vi "oa_Calculate Grid Lines for Cascade Plot.vi"(6 "Y scale":cluster{"offset":dbl, "multiplier":dbl} {"multiplier" format="%.2f"; "offset" format="%.2f"}, 7 "max x axis value":dbl, 8 "order":dbl, 9 "data":dbl[](array[numeric]), 10 "multiplier":dbl, 11 "start index":dbl) -> (3 "output grid lines":cluster{"offset":dbl, dbl, dbl[]})   [LabVIEW 2017]
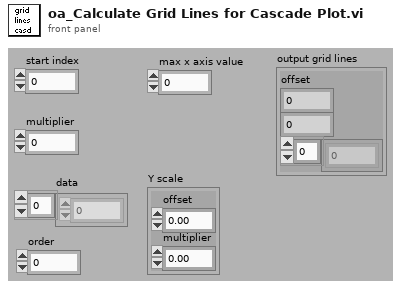
[diagram p1: front panel]
types:
  T1 = cluster{"start index":dbl, "multiplier":dbl, "data":dbl[]}
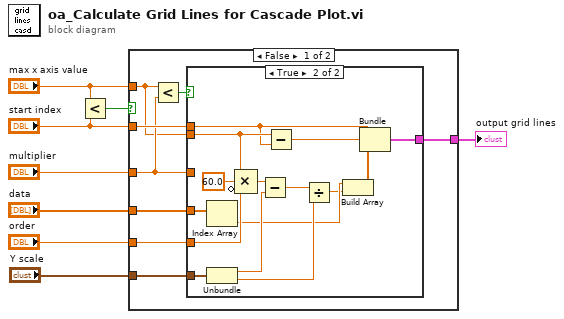
[diagram p0: block diagram]
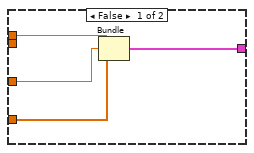
[diagram p2: hidden frame]
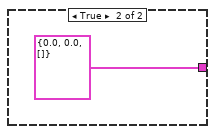
[diagram p3: hidden frame]
diagram:
  n1 = Less?(x="max x axis value", y="start index") -> (x < y?=w8:bool)
  n2 = case shown="False" w8 {
    tunnel: "max x axis value" -> [w12 _]
    tunnel: "start index" -> [w15 _]
    tunnel: "data" -> [w13 _]
    tunnel: "multiplier" -> [w14 _]
    tunnel: [w10 T1 {"start index"=0.0, "multiplier"=0.0, "data"=[]}] -> w3
    tunnel: "order" -> [w11 _]
    tunnel: "Y scale" -> [w9 _]
    frame False {
      n3 = Less?(x=w12, y=w14) -> (x < y?=w16:bool)
      n4 = case shown="True" w16 {
        tunnel: w15 -> [w20 w23]
        tunnel: w14 -> [w19 _]
        tunnel: w13 -> [w18 w32]
        tunnel: w12 -> [_ w24]
        tunnel: w11 -> [_ w34]
        tunnel: [w17 w33] -> w10
        tunnel: w9 -> [_ w30]
        frame False {
          n5 = Bundle("start index"=w20, "multiplier"=w19, "data"=w18) -> (w17:T1)  [unwired: 1 in]
        }
        frame True {
          n6 = Index Array(array=w32) -> (element=w27:dbl)  [unwired: 1 in]
          n7 = Unbundle(w30) -> ("offset"=w29:dbl, "multiplier"=w28:dbl)
          n8 = Compound Arithmetic op=MULTIPLY(w24, 60.0 ("value"), invert w34) -> (w31:dbl)
          n9 = Subtract(x=w31, y=w29) -> (x-y=w25:dbl)
          n10 = Subtract(x=w24, y=w23) -> (x-y=w26:dbl)
          n11 = Divide(x=w25, y=w28) -> (x/y=w22:dbl)
          n12 = Build Array(w27, w22) -> (w21:dbl[])
          n13 = Bundle("start index"=w23, w26, w21) -> (w33:cluster{"start index":dbl, dbl, dbl[]})  [unwired: 1 in]
        }
      }
    }
    frame True {
    }
  }
  "output grid lines" <- w3
